vi "传递波形全局变量.vi"() -> ()   [LabVIEW 2010]
panel:
  in  "波形数据":dbl format="%.2f"
  in  "停止":bool
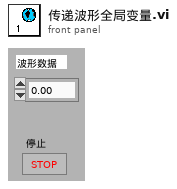
[diagram p1: front panel]
diagram:
